vi "Create MenuItem.vi"(4 "error in (no error)":errorcluster, 5 "Enabled":bool=TRUE, 6 "Item Tag":string, 7 "Item Text":string) -> (0 "error out":errorcluster, 3 "MenuItem out":refnum<k24>)   [LabVIEW 2020, in "NotifyIcon.lvlib"]
uses:
  NotifyIcon.lvlib
  System.Windows.Forms
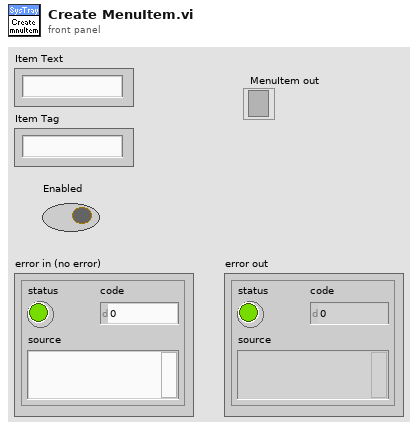
[diagram p1: front panel]
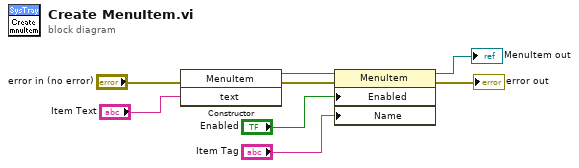
[diagram p0: block diagram]
diagram:
  n1 = constructor class="MenuItem"(error in="error in (no error)", "text"="Item Text") -> (reference out=w3:refnum<k24>, error out=w4:errorcluster)  [unwired: 2 in, 2 out]
  n2 = property class="MenuItem"(reference=w3, error in=w4, "Enabled"="Enabled", "Name"="Item Tag") -> (reference out=→"MenuItem out":refnum<k24>, error out=→"error out":errorcluster)
